vi "2D Helmholtz PDE Solver (Rect Domain).vi"(0 "PDE in":refnum<class "NI_PDE.lvclass">, 11 "error in (no error)":errorcluster) -> (4 "PDE out":refnum<class "NI_PDE.lvclass">, 6 "U(x, y)":dbl[][](array[numeric]), 15 "error out":errorcluster)   [LabVIEW 2020, in "NI_PDE.lvlib"]
doc: "Solves a partial differential equation. You must manually select the polymorphic instance to use."
uses:
  <vilib>/gmath/NI_PDE.lvlib
  <vilib>/gmath/pde.llb/PDEClass/NI_PDE.lvclass
  <vilib>/gmath/pde.llb/PDEClass/PDE_Helmholtz_2D/NI_PDE_Helmholtz_2D.lvclass
  e:/builds/penguin/labview/branches/2020/dev/dist/vi.lib/gmath/pde.llb/PDEClass/NI_PDE.lvclass
  <vilib>/gmath/pde.llb/DomainClass/Domain_Steady_2D_Rect/NI_Domain_Steady_2D_Rect.lvclass
  e:/builds/penguin/labview/branches/2020/dev/dist/vi.lib/gmath/pde.llb/DomainClass/NI_Domain.lvclass
  <vilib>/gmath/pde.llb/BCClass/BC_Steady_2D_Numeric/NI_BC_Steady_2D_Numeric.lvclass
  e:/builds/penguin/labview/branches/2020/dev/dist/vi.lib/gmath/pde.llb/BCClass/NI_BC.lvclass
  <vilib>/gmath/pde.llb/RHSClass/RHS_2D_Numeric/NI_RHS_2D_Numeric.lvclass
  e:/builds/penguin/labview/branches/2020/dev/dist/vi.lib/gmath/pde.llb/RHSClass/NI_RHS.lvclass
  <vilib>/gmath/pde.llb/DomainClass/Domain_Steady_2D_Rect/Domain Data.ctl
  <vilib>/gmath/pde.llb/PDEClass/PDE_2ndOrder_ConstPara/Para Data.ctl
  <vilib>/gmath/pde.llb/PDEClass/PDE Data_Class.ctl
  <vilib>/gmath/pde.llb/RHSClass/NI_RHS.lvclass
  <vilib>/gmath/pde.llb/DomainClass/NI_Domain.lvclass
  <vilib>/gmath/pde.llb/BCClass/NI_BC.lvclass
  <vilib>/gmath/pde.llb/ICClass/NI_IC.lvclass
  <vilib>/gmath/pde.llb/BCClass/BC_Steady_2D_Numeric/BC Data.ctl
  <vilib>/gmath/pde.llb/Common/PDE_BC Type.ctl
  <vilib>/gmath/pde.llb/Common/PDE_BC Position 2D.ctl
  <vilib>/gmath/pde.llb/PDEClass/PDE_2ndOrder_ConstPara/NI_PDE_2ndOrder_ConstPara.lvclass
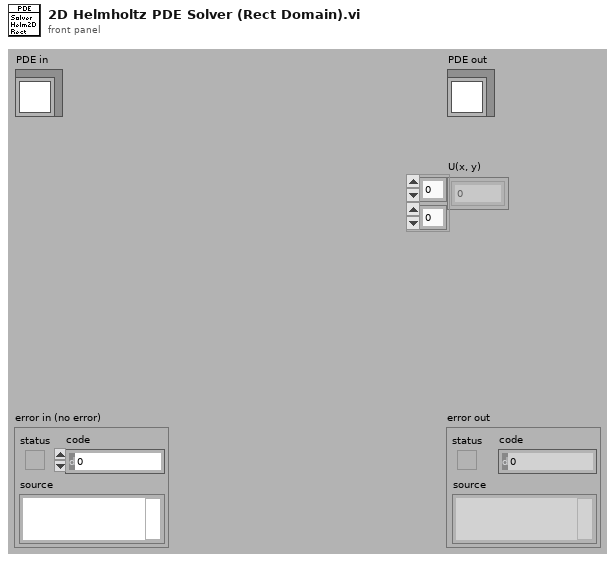
[diagram p1: front panel]
types:
  T1 = typedef "NI_PDE.lvlib/NI_PDE.lvclass/PDE Data_Class.ctl" = cluster{"PDE":refnum<class "NI_PDE.lvclass">, "RHS":refnum<class "NI_RHS.lvclass">, "Domain":refnum<class "NI_Domain.lvclass">, "BC":refnum<class "NI_BC.lvclass">, "IC":refnum<class "NI_IC.lvclass">}
  T2 = typedef "NI_PDE.lvlib/NI_PDE_2ndOrder_ConstPara.lvclass/Para Data.ctl" = cluster{"k":dbl, "a":dbl}
  T3 = typedef "NI_PDE.lvlib/NI_Domain_Steady_2D_Rect.lvclass/Domain Data.ctl" = cluster{"X":cluster{"start x":dbl, "end x":dbl, "# of x-points":i32}, "Y":cluster{"start y":dbl, "end y":dbl, "# of y-points":i32}}
  T4 = typedef "NI_PDE.lvlib/NI_BC_Steady_2D_Numeric.lvclass/BC Data.ctl" = cluster{"type":T5, "position":T6, "G":dbl[]}
  T5 = typedef "NI_PDE.lvlib/PDE_BC Type.ctl" = i32
  T6 = typedef "NI_PDE.lvlib/PDE_BC Position 2D.ctl" = i32
  T7 = typedef "NI_PDE.lvlib/NI_PDE.lvclass/PDE Data_Variant.ctl" = cluster{"parameter":variant, "RHS":variant, "domain":variant, "BC Array":variant[], "IC Array":variant[]}
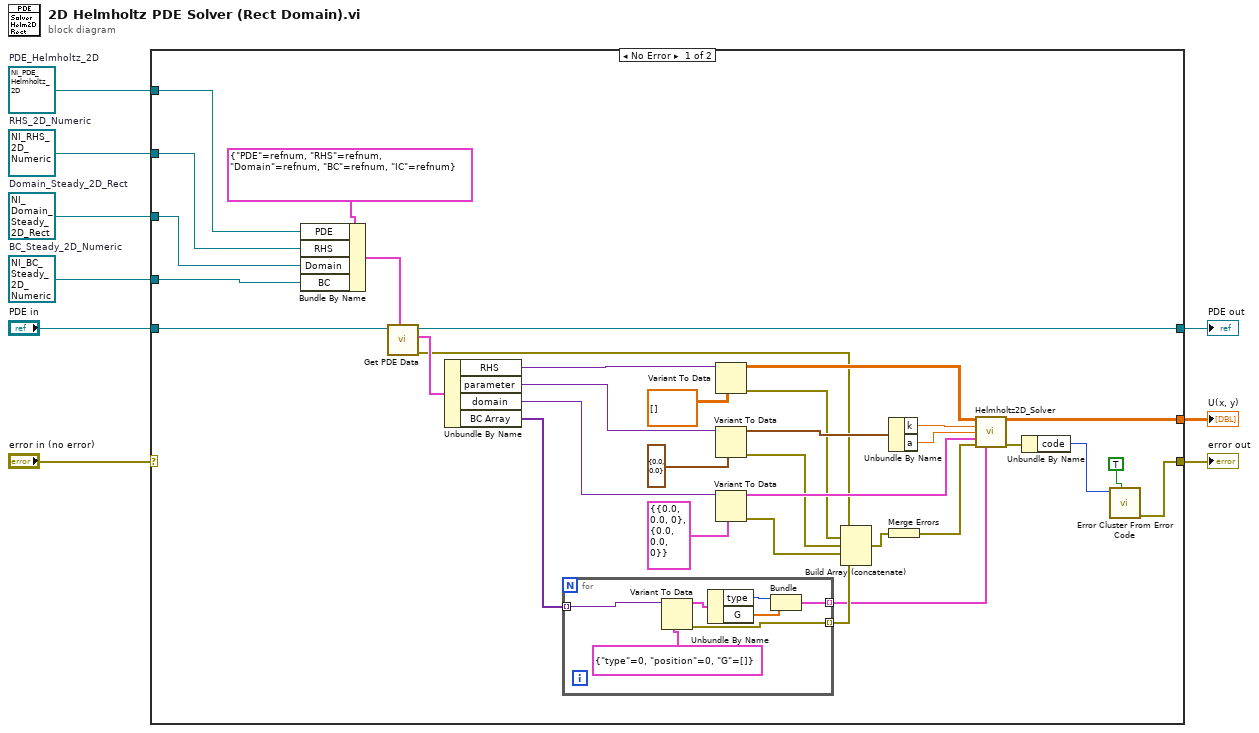
[diagram p0: block diagram]
diagram:
  w1 = refnum<class "NI_RHS_2D_Numeric.lvclass"> refnum  # RHS_2D_Numeric
  w2 = refnum<class "NI_BC_Steady_2D_Numeric.lvclass"> refnum  # BC_Steady_2D_Numeric
  w3 = refnum<class "NI_Domain_Steady_2D_Rect.lvclass"> refnum  # Domain_Steady_2D_Rect
  w4 = refnum<class "NI_PDE_Helmholtz_2D.lvclass"> refnum  # PDE_Helmholtz_2D
  n1 = case shown="No Error" "error in (no error)" {
    selector: "error in (no error)" -> [_ w51]
    tunnel: [w43 _] -> w9
    tunnel: "PDE in" -> [w23 w52]
    tunnel: [w22 w52] -> w7
    tunnel: [w39 w51] -> w6
    tunnel: w4 -> [w14 _]
    tunnel: w3 -> [w12 _]
    tunnel: w2 -> [w11 _]
    tunnel: w1 -> [w13 _]
    frame No Error {
      n2 = Bundle By Name(cluster=T1 {"PDE"=refnum, "RHS"=refnum, "Domain"=refnum, "BC"=refnum, "IC"=refnum} ("target class"), "PDE"=w14, "RHS"=w13, "Domain"=w12, "BC"=w11) -> (w10:T1)
      n3 = call <vilib>:"Get PDE Data.vi"("target class"=w10, "PDE in"=w23) -> ("error out"=w16:errorcluster, "PDE data"=w21:T7, "PDE out"=w22:refnum<class "NI_PDE.lvclass">)  [unwired: 3 in, 4 out]
      n4 = Unbundle By Name(w21) -> ("RHS"=w19:variant, "parameter"=w20:variant, "domain"=w18:variant, "BC Array"=w17:variant[])
      n5 = for {
        tunnel: w17 -> [w49] mode=indexing
        tunnel: [w50] -> w27 mode=indexing
        tunnel: [w45] -> w24 mode=indexing
        n6 = Variant To Data(type=T4 {"type"=0, "position"=0, "G"=[]} ("BC data"), Variant=w49) -> (data=w48:T4, error out=w50:errorcluster)  [unwired: 1 in]
        n7 = Unbundle By Name(w48) -> ("type"=w47:T5, "G"=w46:dbl[])
        n8 = Bundle("type"=w47, "G"=w46) -> (w45:cluster{"type":T5, "G":dbl[]})  [unwired: 1 out]
      }
      n9 = Variant To Data(type=dbl[][] [] ("F(x, y)"), Variant=w19) -> (data=w31:dbl[][], error out=w30:errorcluster)  [unwired: 1 in]
      n10 = Variant To Data(type=T2 {"k"=0.0, "a"=0.0} ("para data"), Variant=w20) -> (data=w35:T2, error out=w29:errorcluster)  [unwired: 1 in]
      n11 = Variant To Data(type=T3 {"X"={"start x"=0.0, "end x"=0.0, "# of x-points"=0}, "Y"={"start y"=0.0, "end y"=0.0, "# of y-points"=0}} ("domain data"), Variant=w18) -> (data=w37:T3, error out=w28:errorcluster)  [unwired: 1 in]
      n12 = Build Array (concatenate)(w16, w30, w29, w28, w27) -> (w26:errorcluster[])
      n13 = Unbundle By Name(w35) -> ("k"=w34:dbl, "a"=w33:dbl)
      n14 = Merge Errors(w26) -> (w25:errorcluster)
      n15 = call <vilib>:"Helmholtz2D_Solver.vi"("F(x, y)"=w31, "k"=w34, "a"=w33, "Domain"=w37, "error in (no error)"=w25, "Boundary Condition"=w24) -> ("U(x, y)"=w43:dbl[][], "error out"=w40:errorcluster)  [unwired: 8 out]
      n16 = Unbundle By Name(w40) -> ("code"=w42:i32)
      n17 = call <vilib>:"Error Cluster From Error Code.vi"("show call chain? (False)"=TRUE, "error code (0)"=w42) -> ("error out"=w39:errorcluster)  [unwired: 1 in, 6 out]
    }
    frame Error {
    }
  }
  "U(x, y)" <- w9
  "error out" <- w6
  "PDE out" <- w7
